vi "Rational Resample.vi"   [LabVIEW 2020, in "NI_AALPro.lvlib"]
doc: "Resamples the input signal <B>X</B> by interpolating <B>X</B>, passing the interpolated signal through an FIR filter, and decimating the filtered signal. Wire data to the <B>X</B> input to determine the polymorphic instance to use or manually select the instance."
uses:
  <vilib>/Analysis/NI_AALPro.lvlib
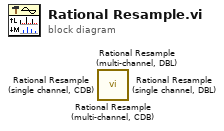
[diagram p0: block diagram]
diagram:
  n1 = call <vilib>:"Rational Resample (multi-channel, CDB).vi"() -> ()  [unwired: 9 in, 3 out]
  n2 = call <vilib>:"Rational Resample (multi-channel, DBL).vi"() -> ()  [unwired: 9 in, 3 out]
  n3 = call <vilib>:"Rational Resample (single channel, CDB).vi"() -> ()  [unwired: 9 in, 3 out]
  n4 = call <vilib>:"Rational Resample (single channel, DBL).vi"() -> ()  [unwired: 9 in, 3 out]
